vi "Acquire Data.vi"(8 "error in (no error)":errorcluster, 11 "Simulated Force Sensor in":refnum<class "Simulated Force Sensor.lvclass">) -> (0 "error out":errorcluster, 3 "Simulated Force Sensor out":refnum<class "Simulated Force Sensor.lvclass">)   [LabVIEW 2020, in "Simulated Force Sensor.lvclass"]
uses:
  Simulated Force Sensor.lvclass
  C:/Users/jharw/Documents/1 Folder to Rule them All/UMD/Inflation-Apparatus/src/Hardware/General Hardware.lvclass
  C:/Users/jharw/Documents/1 Folder to Rule them All/UMD/Inflation-Apparatus/src/Hardware/Sensors/Force Sensors/Force Sensor.lvclass
  General Hardware.lvclass/General Hardware.ctl
  Force Sensor.lvclass/Force Sensor.ctl
  Force Sensor.lvclass
  General Hardware.lvclass
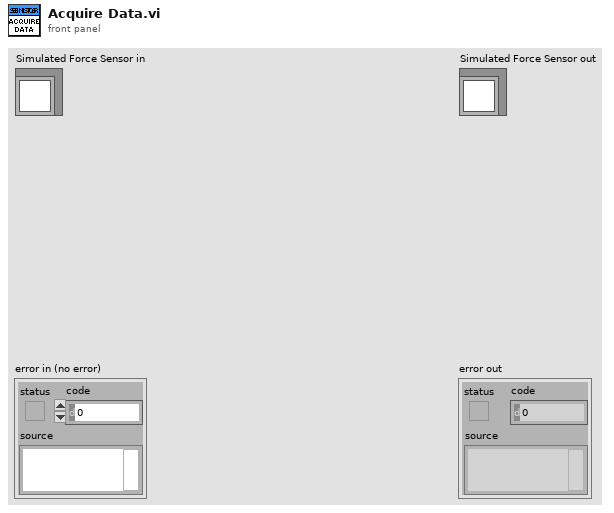
[diagram p1: front panel]
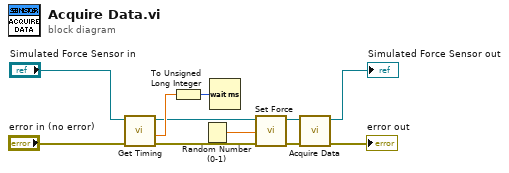
[diagram p0: block diagram]
diagram:
  n1 = call "Get Timing.vi"("error in (no error)"="error in (no error)", "General Hardware in"="Simulated Force Sensor in") -> ("error out"=w7:errorcluster, "time delay (ms)"=w8:dbl, "General Hardware out"=w5:refnum<class "Simulated Force Sensor.lvclass">)  [unwired: 6 in, 1 out]
  n2 = To Unsigned Long Integer(number=w8) -> (unsigned 32bit integer=w9:u32)
  n3 = Random Number (0-1)() -> (number: 0 to 1=w6:dbl)
  n4 = Wait (ms)(milliseconds to wait=w9) -> ()  [unwired: 1 out]
  n5 = call "Set Force.vi"("error in (no error)"=w7, "force (V)"=w6, "Force Sensor in"=w5) -> ("error out"=w3:errorcluster, "Force Sensor out"=w4:refnum<class "Simulated Force Sensor.lvclass">)  [unwired: 7 in]
  n6 = call-parent "Acquire Data.vi"("error in (no error)"=w3, "Force Sensor in"=w4) -> ("error out"=→"error out":errorcluster, "Force Sensor out"=→"Simulated Force Sensor out":refnum<class "Simulated Force Sensor.lvclass">)  [unwired: 8 in]
